vi "Limit20Characters.vi"(11 "trimmed string in":string) -> (3 "trimmed string out":string)   [LabVIEW 2016]
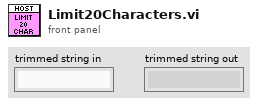
[diagram p1: front panel]
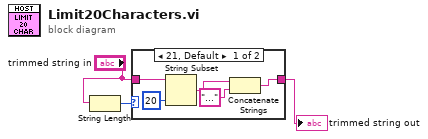
[diagram p0: block diagram]
diagram:
  n1 = String Length(string="trimmed string in") -> (length=w2:i32)
  n2 = case shown="21, Default" w2 {
    tunnel: "trimmed string in" -> [w8 w9]
    tunnel: [w5 w9] -> w1
    frame 21, Default {
      n3 = String Subset(string=w8, length (rest)=20 ("length (rest)")) -> (substring=w6:string)  [unwired: 1 in]
      n4 = Concatenate Strings(w6, "..." ("string")) -> (w5:string)
    }
    frame 0..20 {
    }
  }
  "trimmed string out" <- w1
